vi "UDT_application_RawStringtoCluster.vi"() -> (3 "Unit Test Framework Results":T1)   [LabVIEW 2017]
doc: "Use this template to create a user-defined test VI. Define your test requirements and wire the results to the <b>Result (Test)</b> control. Do not modify the <b>Unit Test Framework Results</b> indicator."
uses:
  <vilib>/utf/common/utf_test_result_troll.ctl
  <vilib>/utf/common/utf_test_result.ctl
  <vilib>/utf/common/utf_test_result_failure.ctl
  <vilib>/utf/common/utf_test_comparison_operators.ctl
  <vilib>/utf/common/utf_vi_tag.ctl
  <vilib>/Control Software Solutions Ltd/UTF Helper/SubVIs/UTF Double Equals.vi
  <vilib>/Control Software Solutions Ltd/UTF Helper/SubVIs/UTF Boolean Equals.vi
  <vilib>/Control Software Solutions Ltd/UTF Helper/Unit Test Helper.lvlib
  <vilib>/utf/NI_UnitTestFramework.lvlib
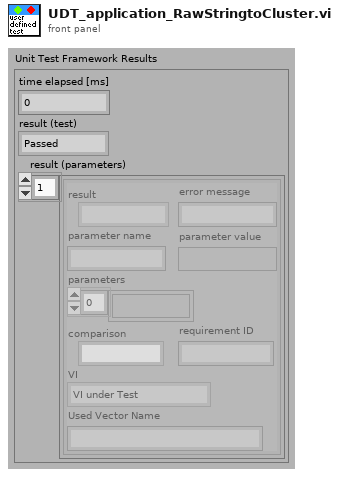
[diagram p1: front panel]
types:
  T1 = typedef "NI_UnitTestFramework.lvlib/utf_test_result_troll.ctl" = cluster{"time elapsed [ms]":u32, "result (test)":T2, "result (parameters)":T3[]}
  T2 = typedef "NI_UnitTestFramework.lvlib/utf_test_result.ctl" = enum16{"Passed", "Failed", "Error", "Skipped", "Not Processed"}
  T3 = typedef "NI_UnitTestFramework.lvlib/utf_test_result_failure.ctl" = cluster{"result":T2, "error message":string, "parameter name":string, "parameter value":variant, "parameters":variant[], "comparison":T4, "requirement ID":string, "VI":T5, "Used Vector Name":string}
  T4 = typedef "NI_UnitTestFramework.lvlib/utf_test_comparison_operators.ctl" = enum16{"=", "!=", ">", ">=", "<", "<=", "range", "symmetric tolerance", "asymmetric tolerance", "string contains", "string not contain", "array size", "string length", "array range", "by element", "array range (limit array)", "user-defined", "array contains", "array not contain", "vector length", "= (elm)", "!= (elm)", "= (case insensitive)", "!= (case insensitive)"}
  T5 = typedef "NI_UnitTestFramework.lvlib/utf_vi_tag.ctl" = enum16{"Setup VI", "VI under Test", "Teardown VI"}
  T6 = typedef "dataIn.ctl" = cluster{"Xtarget":dbl, "Ytarget":dbl, "Ztarget":dbl, "X_Attractor 1":dbl, "Y_Attractor 1":dbl, "Z_Attractor 1":dbl, "X_Attractor 2":dbl, "Y_Attractor 2":dbl, "Z_Attractor 2":dbl, "Traj Flag":bool, "DeadZone":dbl, "Assistance":bool, "Shutdown?":bool, "AssistanceLevel":dbl}
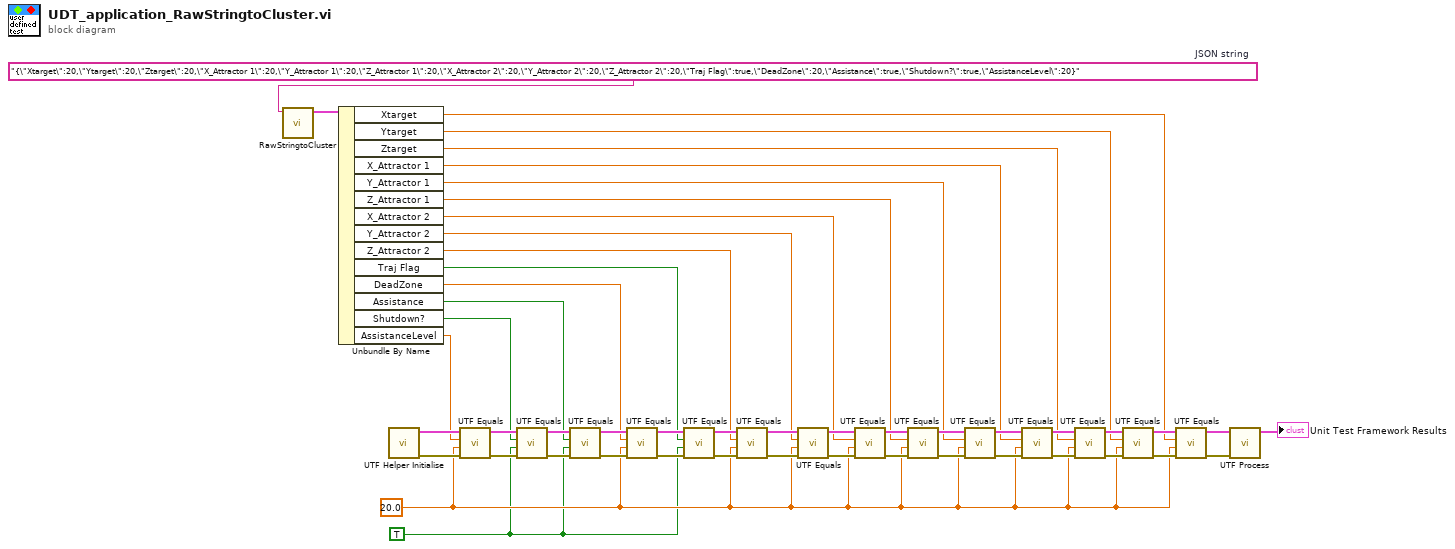
[diagram p0: block diagram]
diagram:
  w1 = "{\"Xtarget\":20,\"Ytarget\":20,\"Ztarget\":20,\"X_Attractor 1\":20,\"Y_Attractor 1\":20,\"Z_Attractor 1\":20,\"X_Attractor 2\":20,\"Y_Attractor 2\":20,\"Z_Attractor 2\":20,\"Traj Flag\":true,\"DeadZone\":20,\"Assistance\":true,\"Shutdown?\":true,\"AssistanceLevel\":20}"  # JSON string
  w2 = TRUE ("Test Value")
  w3 = 20.0 ("Xtarget")
  n1 = call "RawStringtoCluster.vi"("Raw String"=w1) -> ("DataIn"=w42:T6)  [unwired: 9 in, 1 out]
  n2 = Unbundle By Name(w42) -> ("Xtarget"=w4:dbl, "Ytarget"=w5:dbl, "Ztarget"=w12:dbl, "X_Attractor 1"=w13:dbl, "Y_Attractor 1"=w14:dbl, "Z_Attractor 1"=w15:dbl, "X_Attractor 2"=w16:dbl, "Y_Attractor 2"=w17:dbl, "Z_Attractor 2"=w30:dbl, "Traj Flag"=w31:bool, "DeadZone"=w32:dbl, "Assistance"=w39:bool, "Shutdown?"=w40:bool, "AssistanceLevel"=w41:dbl)
  n3 = call <vilib>:"UTF Helper Initialise.vi"() -> ("error out"=w45:errorcluster, "results array"=w46:T3[])  [unwired: 10 in]
  n4 = call-poly <vilib>:"UTF Equals.vi"("error in (no error)"=w45, "Test Value"=w3, "Input"=w41, "Input Results"=w46) -> ("error out"=w44:errorcluster, "Output Results"=w47:T3[])  [unwired: 6 in]
  n5 = call-poly <vilib>:"UTF Equals.vi"("error in (no error)"=w44, "Test Value"=w2, "Input"=w40, "Input Results"=w47) -> ("error out"=w43:errorcluster, "Output Results"=w48:T3[])  [unwired: 6 in]
  n6 = call-poly <vilib>:"UTF Equals.vi"("error in (no error)"=w43, "Test Value"=w2, "Input"=w39, "Input Results"=w48) -> ("error out"=w38:errorcluster, "Output Results"=w37:T3[])  [unwired: 6 in]
  n7 = call-poly <vilib>:"UTF Equals.vi"("error in (no error)"=w38, "Test Value"=w3, "Input"=w32, "Input Results"=w37) -> ("error out"=w33:errorcluster, "Output Results"=w36:T3[])  [unwired: 6 in]
  n8 = call-poly <vilib>:"UTF Equals.vi"("error in (no error)"=w33, "Test Value"=w2, "Input"=w31, "Input Results"=w36) -> ("error out"=w34:errorcluster, "Output Results"=w35:T3[])  [unwired: 6 in]
  n9 = call-poly <vilib>:"UTF Equals.vi"("error in (no error)"=w34, "Test Value"=w3, "Input"=w30, "Input Results"=w35) -> ("error out"=w29:errorcluster, "Output Results"=w28:T3[])  [unwired: 6 in]
  n10 = call-poly <vilib>:"UTF Equals.vi"("error in (no error)"=w29, "Test Value"=w3, "Input"=w17, "Input Results"=w28) -> ("error out"=w27:errorcluster, "Output Results"=w18:T3[])  [unwired: 6 in]
  n11 = call-poly <vilib>:"UTF Equals.vi"("error in (no error)"=w27, "Test Value"=w3, "Input"=w16, "Input Results"=w18) -> ("error out"=w26:errorcluster, "Output Results"=w19:T3[])  [unwired: 6 in]
  n12 = call-poly <vilib>:"UTF Equals.vi"("error in (no error)"=w26, "Test Value"=w3, "Input"=w15, "Input Results"=w19) -> ("error out"=w25:errorcluster, "Output Results"=w20:T3[])  [unwired: 6 in]
  n13 = call-poly <vilib>:"UTF Equals.vi"("error in (no error)"=w25, "Test Value"=w3, "Input"=w14, "Input Results"=w20) -> ("error out"=w24:errorcluster, "Output Results"=w21:T3[])  [unwired: 6 in]
  n14 = call-poly <vilib>:"UTF Equals.vi"("error in (no error)"=w24, "Test Value"=w3, "Input"=w13, "Input Results"=w21) -> ("error out"=w23:errorcluster, "Output Results"=w22:T3[])  [unwired: 6 in]
  n15 = call-poly <vilib>:"UTF Equals.vi"("error in (no error)"=w23, "Test Value"=w3, "Input"=w12, "Input Results"=w22) -> ("error out"=w11:errorcluster, "Output Results"=w10:T3[])  [unwired: 6 in]
  n16 = call-poly <vilib>:"UTF Equals.vi"("error in (no error)"=w11, "Test Value"=w3, "Input"=w5, "Input Results"=w10) -> ("error out"=w8:errorcluster, "Output Results"=w9:T3[])  [unwired: 6 in]
  n17 = call-poly <vilib>:"UTF Equals.vi"("error in (no error)"=w8, "Test Value"=w3, "Input"=w4, "Input Results"=w9) -> ("error out"=w6:errorcluster, "Output Results"=w7:T3[])  [unwired: 6 in]
  n18 = call <vilib>:"UTF Process.vi"("error in (no error)"=w6, "results array"=w7) -> ("Unit Test Framework Results"=→"Unit Test Framework Results":T1)  [unwired: 9 in]
